vi "Script Matlab (SubVI).vi"(7 "Color 3":u32, 8 "error in (no error)":errorcluster, 9 "Color 2":u32, 10 "Color":u32, 11 "name":string) -> (0 "error out":errorcluster, 3 "String":string)   [LabVIEW 2015]
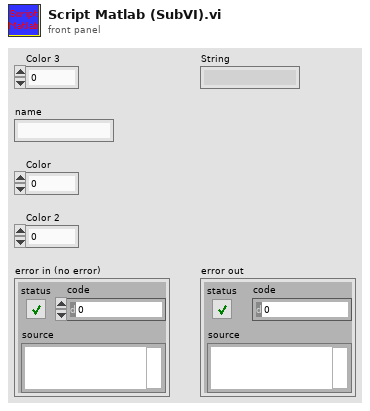
[diagram p1: front panel]
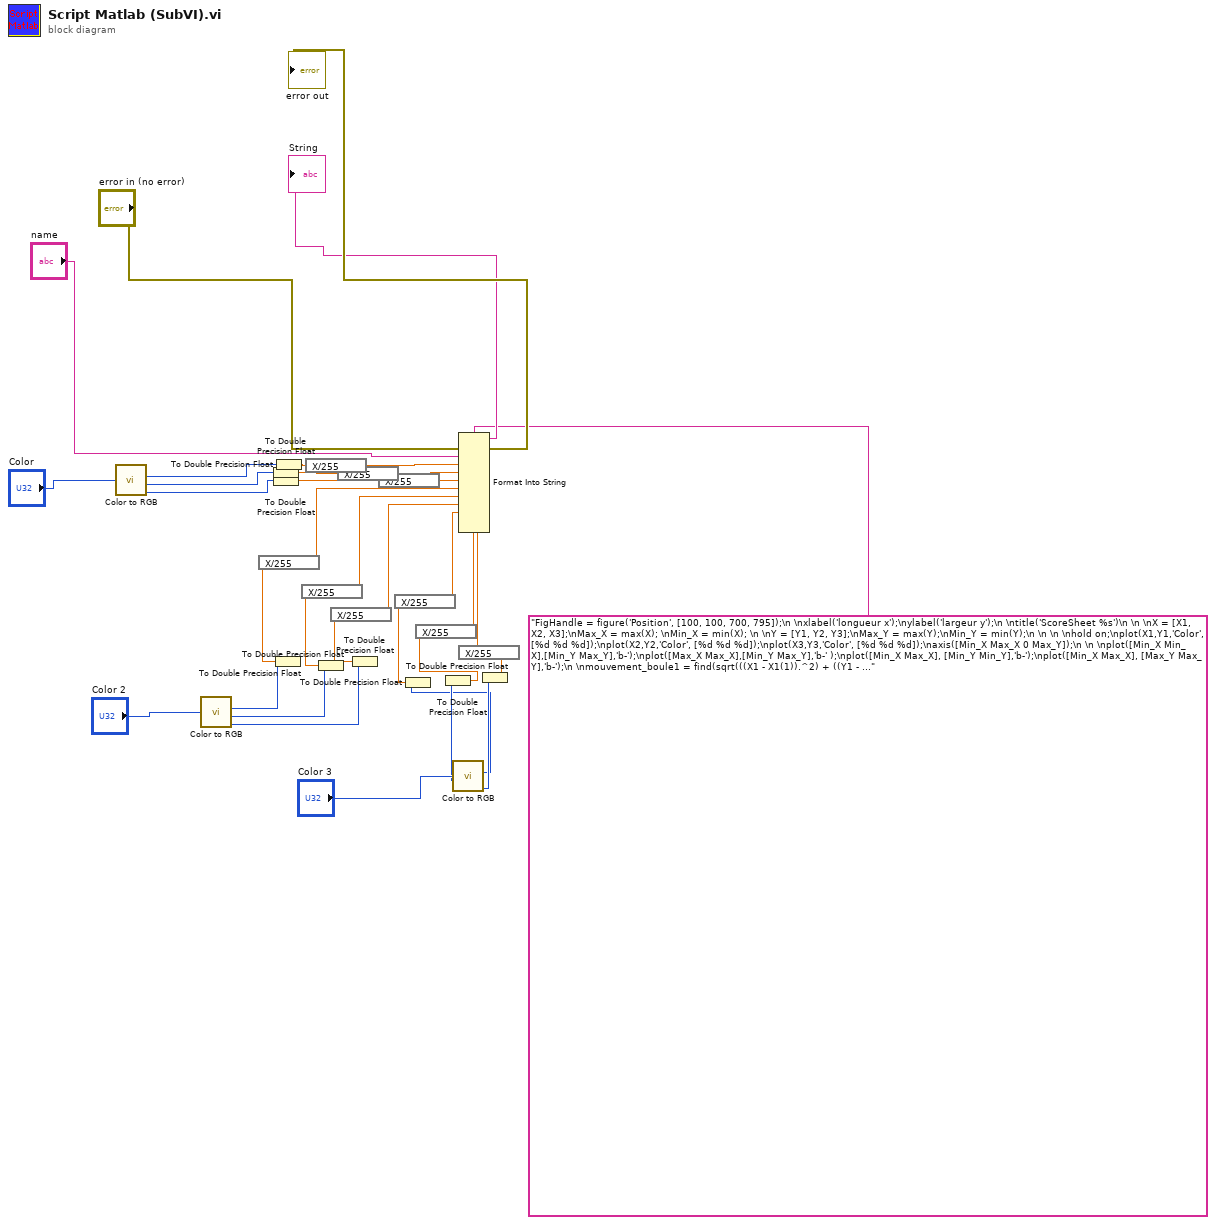
[diagram p0: block diagram]
diagram:
  n1 = call <vilib>:"Color to RGB.vi"("Color"="Color") -> ("R"=w2:u8, "G"=w3:u8, "B"=w4:u8)  [unwired: 1 out]
  n2 = call <vilib>:"Color to RGB.vi"("Color"="Color 2") -> ("R"=w5:u8, "G"=w6:u8, "B"=w7:u8)  [unwired: 1 out]
  n3 = To Double Precision Float(number=w3) -> (double precision float=w9:dbl)
  n4 = To Double Precision Float(number=w4) -> (double precision float=w10:dbl)
  n5 = To Double Precision Float(number=w5) -> (double precision float=w11:dbl)
  n6 = expression code="X/255"(w11) -> (w17:dbl)
  n7 = To Double Precision Float(number=w2) -> (double precision float=w8:dbl)
  n8 = expression code="X/255"(w8) -> (w14:dbl)
  n9 = To Double Precision Float(number=w6) -> (double precision float=w12:dbl)
  n10 = expression code="X/255"(w12) -> (w18:dbl)
  n11 = expression code="X/255"(w9) -> (w15:dbl)
  n12 = To Double Precision Float(number=w7) -> (double precision float=w13:dbl)
  n13 = expression code="X/255"(w13) -> (w19:dbl)
  n14 = expression code="X/255"(w10) -> (w16:dbl)
  n15 = call <vilib>:"Color to RGB.vi"("Color"="Color 3") -> ("R"=w20:u8, "G"=w21:u8, "B"=w22:u8)  [unwired: 1 out]
  n16 = To Double Precision Float(number=w20) -> (double precision float=w23:dbl)
  n17 = expression code="X/255"(w23) -> (w26:dbl)
  n18 = To Double Precision Float(number=w21) -> (double precision float=w24:dbl)
  n19 = expression code="X/255"(w24) -> (w27:dbl)
  n20 = To Double Precision Float(number=w22) -> (double precision float=w25:dbl)
  n21 = expression code="X/255"(w25) -> (w28:dbl)
  n22 = Format Into String(format string="FigHandle = figure('Position', [100, 100, 700, 795]);\n \nxlabel('longueur x');\nylabel('largeur y');\n \ntitle('ScoreSheet %s')\n \n \nX = [X1, X2, X3];\nMax_X = max(X); \nMin_X = min(X); \n \nY = [Y1, Y2, Y3];\nMax_Y = max(Y);\nMin_Y = min(Y);\n \n \n \nhold on;\nplot(X1,Y1,'Color', [%d %d %d]);\nplot(X2,Y2,'Color', [%d %d %d]);\nplot(X3,Y3,'Color', [%d %d %d]);\naxis([Min_X Max_X 0 Max_Y]);\n \n \nplot([Min_X Min_X],[Min_Y Max_Y],'b-');\nplot([Max_X Max_X],[Min_Y Max_Y],'b-' );\nplot([Min_X Max_X], [Min_Y Min_Y],'b-');\nplot([Min_X Max_X], [Max_Y Max_Y],'b-');\n \nmouvement_boule1 = find(sqrt(((X1 - X1(1)).^2) + ((Y1 - Y1(1)).^2)) > 2);\nmouvement_boule2 = find(sqrt(((X2 - X2(1)).^2) + ((Y2 - Y2(1)).^2)) > 2);\nmouvement_boule3 = find(sqrt(((X3 - X3(1)).^2) + ((Y3 - Y3(1)).^2)) > 2);\n\n \n \nTrois_boules_bougent = 0;\nAucune_boule_bouge = 0;\nUne_boule_bouge = 0;\nDeux_boules_bougent = 0;\n \n \nif (length(mouvement_boule1) > 1 && length(mouvement_boule3) > 1 && length(mouvement_boule2) > 1)\n text(200, 35, 'Nombre de boules touchees: 2');\n Trois_boules_bougent = 1;\nelseif (isempty(mouvement_boule1) && isempty(mouvement_boule2) && isempty(mouvement_boule1))\n text(200, 35, 'Aucune boule n a bouge');\n Aucune_boule_bouge = 1;\nelseif ((length(mouvement_boule1) > 1 && length(mouvement_boule2) > 1) || (length(mouvement_boule1) > 1 && length(mouvement_boule3) > 1) || (length(mouvement_boule2) > 1 && length(mouvement_boule3) > 1)) \n text(200, 35, 'Nombre de boules touchees: 1');\n Deux_boules_bougent = 1;\nelse\n text(200, 35, 'Nombre de boules touchees: 0');\n Une_boule_bouge = 1;\nend\n \n \n \nBoule1_1 = 0;\nBoule1_2 = 0;\nBoule1_3 = 0;\nBoule2_1 = 0;\nBoule2_2 = 0;\nBoule2_3 = 0;\nBoule3_1 = 0;\nBoule3_2 = 0;\nBoule3_3 = 0;\n \nif (Trois_boules_bougent)\n \n if (mouvement_boule1(1) < mouvement_boule2(1) && mouvement_boule1(1) < mouvement_boule3(1))\n Boule1_1 = 1;\n if (mouvement_boule2(1) < mouvement_boule3(1))\n Boule2_2 = 1;\n Boule3_3 = 1;\n else\nBoule3_2 = 1;\n Boule2_3 = 1;\n end\n elseif (mouvement_boule2(1) < mouvement_boule1(1) && mouvement_boule2(1) < mouvement_boule3(1))\n Boule2_1 = 1;\n if (mouvement_boule1(1) < mouvement_boule3(1))\n Boule1_2 = 1;\n Boule3_3 = 1;\n else\n Boule3_2 = 1;\n Boule1_3 = 1;\n end\n elseif (mouvement_boule3(1) < mouvement_boule1(1) && mouvement_boule3(1) < mouvement_boule2(1))\n Boule3_1 = 1;\n if (mouvement_boule1(1) < mouvement_boule2(1))\n Boule1_2 = 1;\n Boule2_3 = 1;\n else\n Boule2_3 = 1;\n Boule1_3 = 1;\n end\n end\nelseif (Deux_boules_bougent)\n  if (isempty(mouvement_boule1))\n if (mouvement_boule2(1) < mouvement_boule3(1))\n Boule2_1 = 1;\n Boule3_2 = 1;\n else\n Boule3_1 = 1;\n Boule2_2 = 1;\n end\n elseif (isempty(mouvement_boule2))\n if (mouvement_boule1(1) < mouvement_boule3(1))\n Boule1_1 = 1;\n Boule3_2 = 1;\n else\n Boule3_1 = 1;\n Boule1_2 = 1;\n end\n elseif (isempty(mouvement_boule3))\n if (mouvement_boule1(1) < mouvement_boule2(1))\n Boule1_1 = 1;\n Boule2_2 = 1;\n else\n Boule2_1 = 1;\n Boule1_2 = 1;\n end\n end \nelseif (Une_boule_bouge)\n if (length(mouvement_boule1))\n text(400, 60, 'la boule 1 a bouge');\n elseif (length(mouvement_boule2))\n text(400, 60, 'la boule 2 a bouge');\n elseif (length(mouvement_boule3))\n text(400, 60, 'la boule 3 a bouge');\n end\nend\n \nif (Boule1_1)\nif (length(mouvement_boule2))\n     plot(X2(mouvement_boule2(1)), Y3(mouvement_boule2(1)), 'bo','MarkerSize',15);\nend\nif (length(mouvement_boule3))\n     plot(X3(mouvement_boule3(1)), Y3(mouvement_boule3(1)), 'bo','MarkerSize',15); \nend\nelseif (Boule2_1)\nif (length(mouvement_boule1)) \n     plot(X1(mouvement_boule1(1)), Y1(mouvement_boule1(1)), 'bo','MarkerSize',15);\nend\nif (length(mouvement_boule3))\n     plot(X3(mouvement_boule3(1)), Y3(mouvement_boule3(1)), 'bo','MarkerSize',15); \nend\nelseif(Boule3_1)\nif (length(mouvement_boule1)) \n     plot(X1(mouvement_boule1(1)), Y1(mouvement_boule1(1)), 'bo','MarkerSize',15);\nend\nif (length(mouvement_boule2))\n     plot(X2(mouvement_boule2(1)), Y3(mouvement_boule2(1)), 'bo','MarkerSize',15);\nend\nend\n\n \nZ = 2;\nrayon_boule = 6;\nTrois_bandes_touchees = [];\n \n if (Boule1_1)\n \nX1_bis = X1(mouvement_boule1(1):end);\n Y1_bis = Y1(mouvement_boule1(1):end);\n \n Bande_droite_boule1 = find((X1_bis + rayon_boule + Z) >= Max_X);\n Bande_gauche_boule1 = find((X1_bis - rayon_boule - Z) <= Min_X);\n Bande_basse_boule1 = find((Y1_bis - rayon_boule - Z) <= Min_Y);\n Bande_haute_boule1 = find((Y1_bis + rayon_boule + Z) >= Max_Y);\n \n idxTouch1 = sort([Bande_droite_boule1, Bande_gauche_boule1, Bande_basse_boule1, Bande_haute_boule1]);\n Contact_bande_boule1 = idxTouch1([1, 1 + find(diff(idxTouch1) > 1)]);\n plot(X1_bis(Contact_bande_boule1), Y1_bis(Contact_bande_boule1), 'ro','MarkerSize',15);\n \n Trois_bandes_touchees = Contact_bande_boule1;\n \n elseif (Boule2_1)\n \nX2_bis = X2(mouvement_boule2(1):end);\nY2_bis = Y2(mouvement_boule2(1):end);\n \n Bande_droite_boule2 = find((X2_bis + rayon_boule + Z) >= Max_X);\n Bande_gauche_boule2 = find((X2_bis - rayon_boule - Z) <= Min_X);\n Bande_basse_boule2 = find((Y2_bis - rayon_boule - Z) <= Min_Y);\n Bande_haute_boule2 = find((Y2_bis + rayon_boule + Z) >= Max_Y);\n \n idxTouch2 = sort([Bande_droite_boule2, Bande_gauche_boule2, Bande_basse_boule2, Bande_haute_boule2]);\n Contact_bande_boule2 = idxTouch2([1, 1 + find(diff(idxTouch2) > 1)]);\n plot(X2_bis(Contact_bande_boule2), Y2_bis(Contact_bande_boule2), 'ro','MarkerSize',15);\n \n Trois_bandes_touchees = Contact_bande_boule2;\n \n elseif (Boule3_1)\n \n X3_bis = X3(mouvement_boule3(1):end);\n Y3_bis = Y3(mouvement_boule3(1):end);\n \n Bande_droite_boule3 = find((X3_bis + rayon_boule + Z) >= Max_X);\n Bande_gauche_boule3 = find((X3_bis - rayon_boule - Z) <= Min_X);\n Bande_basse_boule3 = find((Y3_bis - rayon_boule - Z) <= Min_Y);\n Bande_haute_boule3 = find((Y3_bis + rayon_boule + Z) >= Max_Y);\n \n idxTouch3 = sort([Bande_droite_boule3, Bande_gauche_boule3, Bande_basse_boule3, Bande_haute_boule3]);\n Contact_bande_boule3 = idxTouch3([1, 1 + find(diff(idxTouch3) > 1)]);\n plot(X3_bis(Contact_bande_boule3), Y3_bis(Contact_bande_boule3), 'ro','MarkerSize',15);\n \n Trois_bandes_touchees = Contact_bande_boule3;\n end \n \nTrois_bandes_touchees_bis = [];\n \nif (Trois_boules_bougent)\n if (Boule1_1)\n if (Boule2_2)\n X1_bis = X1(mouvement_boule2(1):mouvement_boule3(1));\n Y1_bis = Y1(mouvement_boule2(1):mouvement_boule3(1));\n \n Bande_droite_boule1 = find((X1_bis + rayon_boule + Z) >= Max_X);\n Bande_gauche_boule1 = find((X1_bis - rayon_boule - Z) <= Min_X);\n Bande_basse_boule1 = find((Y1_bis - rayon_boule - Z) <= Min_Y);\n Bande_haute_boule1 = find((Y1_bis + rayon_boule + Z) >= Max_Y);\n \n idxTouch1 = sort([Bande_droite_boule1, Bande_gauche_boule1, Bande_basse_boule1, Bande_haute_boule1]);\n Contact_bande_boule1 = idxTouch1([1, 1 + find(diff(idxTouch1) > 1)]);\n \n Trois_bandes_touchees_bis = Contact_bande_boule1;\n \n elseif (Boule3_2)\n \n X1_bis = X1(mouvement_boule3(1):mouvement_boule2(1));\n Y1_bis = Y1(mouvement_boule3(1):mouvement_boule2(1));\n \n Bande_droite_boule1 = find((X1_bis + rayon_boule + Z) >= Max_X);\n Bande_gauche_boule1 = find((X1_bis - rayon_boule - Z) <= Min_X);\n Bande_basse_boule1 = find((Y1_bis - rayon_boule - Z) <= Min_Y);\n Bande_haute_boule1 = find((Y1_bis + rayon_boule + Z) >= Max_Y);\n \n idxTouch1 = sort([Bande_droite_boule1, Bande_gauche_boule1, Bande_basse_boule1, Bande_haute_boule1]);\nContact_bande_boule1 = idxTouch1([1, 1 + find(diff(idxTouch1) > 1)]);\n \n Trois_bandes_touchees_bis = Contact_bande_boule1;\n \n end\n elseif (Boule2_1)\n if (Boule1_2)\n \nX2_bis = X2(mouvement_boule1(1):mouvement_boule3(1));\n Y2_bis = Y2(mouvement_boule1(1):mouvement_boule3(1));\n \n Bande_droite_boule2 = find((X2_bis + rayon_boule + Z) >= Max_X);\n Bande_gauche_boule2 = find((X2_bis - rayon_boule - Z) <= Min_X);\n Bande_basse_boule2 = find((Y2_bis - rayon_boule - Z) <= Min_Y);\n Bande_haute_boule2 = find((Y2_bis + rayon_boule + Z) >= Max_Y);\n \n idxTouch2 = sort([Bande_droite_boule2, Bande_gauche_boule2, Bande_basse_boule2, Bande_haute_boule2]);\n Contact_bande_boule2 = idxTouch2([1, 1 + find(diff(idxTouch2) > 1)]);\n \n Trois_bandes_touchees_bis = Contact_bande_boule2;\n \n elseif(Boule3_2)\n \n X2_bis = X2(mouvement_boule3(1):mouvement_boule1(1));\n Y2_bis = Y2(mouvement_boule3(1):mouvement_boule1(1));\n \n Bande_droite_boule2 = find((X2_bis + rayon_boule + Z) >= Max_X);\n Bande_gauche_boule2 = find((X2_bis - rayon_boule - Z) <= Min_X);\n Bande_basse_boule2 = find((Y2_bis - rayon_boule - Z) <= Min_Y);\n Bande_haute_boule2 = find((Y2_bis + rayon_boule + Z) >= Max_Y);\n \n idxTouch2 = sort([Bande_droite_boule2, Bande_gauche_boule2, Bande_basse_boule2, Bande_haute_boule2]);\n Contact_bande_boule2 = idxTouch2([1, 1 + find(diff(idxTouch2) > 1)]);\n \n Trois_bandes_touchees_bis = Contact_bande_boule2;\n \n end\nelseif (Boule3_1)\n if (Boule1_2)\n \n X3_bis = X3(mouvement_boule1(1):mouvement_boule2(1));\n Y3_bis = Y3(mouvement_boule1(1):mouvement_boule2(1));\n \n Bande_droite_boule3 = find((X3_bis + rayon_boule + Z) >= Max_X);\n Bande_gauche_boule3 = find((X3_bis - rayon_boule - Z) <= Min_X);\n Bande_basse_boule3 = find((Y3_bis - rayon_boule - Z) <= Min_Y);\n Bande_haute_boule3 = find((Y3_bis + rayon_boule + Z) >= Max_Y);\n \n idxTouch3 = sort([Bande_droite_boule3, Bande_gauche_boule3, Bande_basse_boule3, Bande_haute_boule3]);\n Contact_bande_boule3 = idxTouch3([1, 1 + find(diff(idxTouch3) > 1)]);\n \n Trois_bandes_touchees_bis = Contact_bande_boule3;\n \n elseif (Boule2_2)\n \n X3_bis = X3(mouvement_boule2(1):mouvement_boule1(1));\n Y3_bis = Y3(mouvement_boule2(1):mouvement_boule1(1));\n \n Bande_droite_boule3 = find((X3_bis + rayon_boule + Z) >= Max_X);\n Bande_gauche_boule3 = find((X3_bis - rayon_boule - Z) <= Min_X);\n Bande_basse_boule3 = find((Y3_bis - rayon_boule - Z) <= Min_Y);\n Bande_haute_boule3 = find((Y3_bis + rayon_boule + Z) >= Max_Y);\n \n idxTouch3 = sort([Bande_droite_boule3, Bande_gauche_boule3, Bande_basse_boule3, Bande_haute_boule3]);\n Contact_bande_boule3 = idxTouch3([1, 1 + find(diff(idxTouch3) > 1)]);\n \n Trois_bandes_touchees_bis = Contact_bande_boule3;\n \nend\nend\nend\n \n FormatSpec=['Number of band(s) touched:' num2str(length(Trois_bandes_touchees))'];\n str1=sprintf(FormatSpec, length(Trois_bandes_touchees));\n text(200,50,str1);\n \n \n if (Boule1_1)\n text(400, 65, 'Score sheet for \"red\"');\n elseif (Boule2_1)\n text(400, 65, 'Score sheet for \"yellow\"');\n elseif (Boule3_1)\n text(400, 65, 'Score sheet for \"white\"');\n end\n \n \nif (length(Trois_bandes_touchees_bis) >= 3 && Trois_boules_bougent)\n text(200, 65, '--Win--')\nelse\n text(200, 65, '--Fail--')\nend\n \nlegend('boule rouge','boule jaune','boule blanche','Location','SouthEast')\nhold off;\npause(20);\nprint('-dpdf','ScoreSheet.pdf')\n", error in="error in (no error)", "name", w14, w15, w16, w17, w18, w19, w26, w27, w28) -> (resulting string=→"String":string, error out=→"error out":errorcluster)  [unwired: 1 in]
